vi "HSSS encode.vi"(10 "Crew Status":bool[](array[boolean]), 11 "Array":dbl[](array[numeric])=[111.12345886230469, 111.12345886230469, 111.12345886230469, 9199.099609375, 9299.2001953125, 9399.5, 9499.599609375, 9599.7001953125, 9699.7998046875, 9799.900390625] format="%#.8g") -> (3 "Power string":string)   [LabVIEW 2021]
panel:
  out "length 3":i32
  out "length 2":i32
  out "length":i32
  in  "Array 2":dbl[](array[numeric])=[0.0, 0.0, 0.0, 0.0, 0.0, 0.0, 0.0, 0.0, 0.0, 0.0]
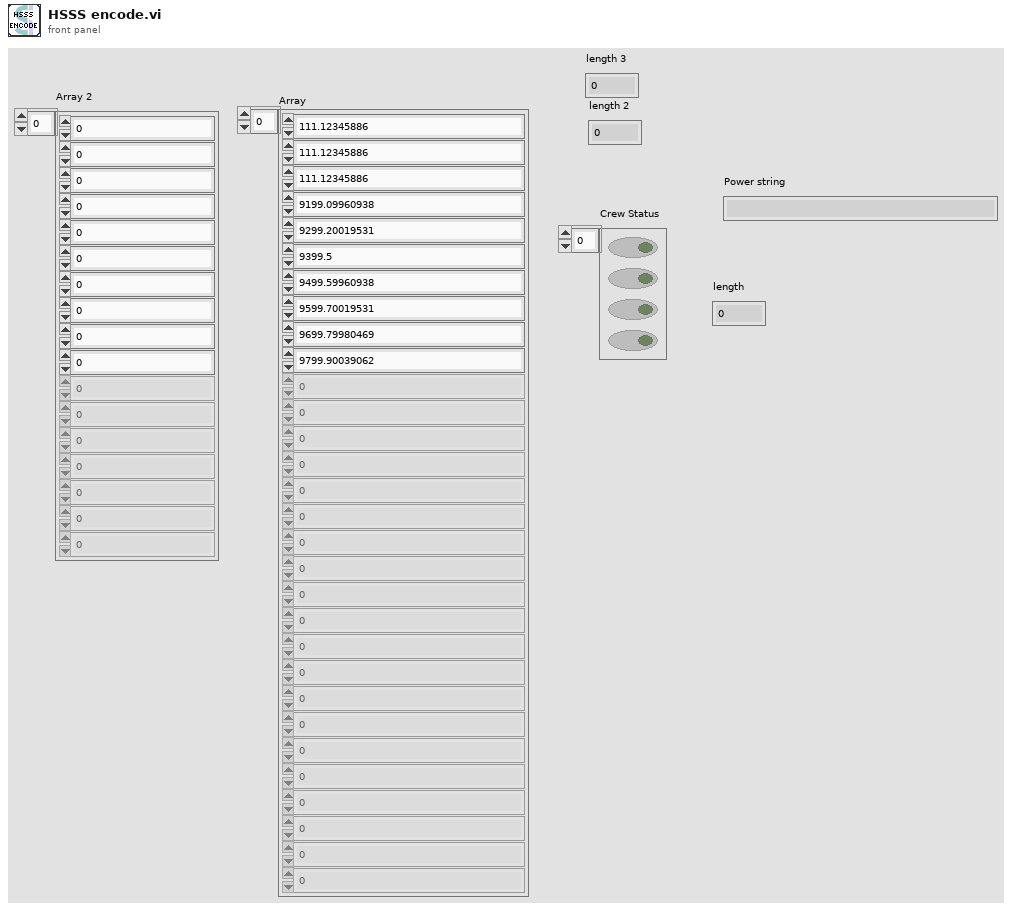
[diagram p1: front panel]
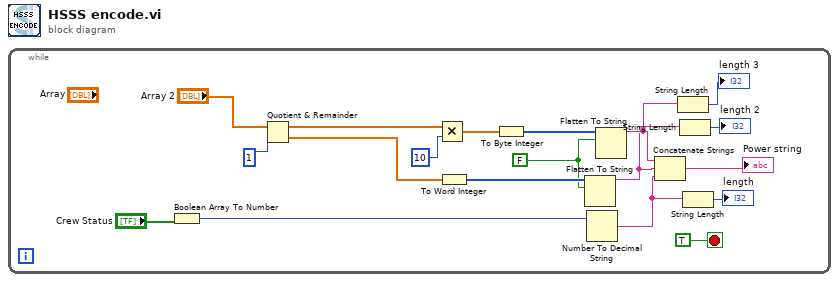
[diagram p0: block diagram]
diagram:
  n1 = while {
    stop <- TRUE stop-if-true
    w11 = FALSE ("prepend array or string size? (T)")
    n2 = Boolean Array To Number(Boolean array="Crew Status") -> (number=w8:u32)
    n3 = Quotient & Remainder(x="Array 2", y=1) -> (x-y*floor(x/y)=w18:dbl[], floor(x/y)=w15:dbl[])
    n4 = Multiply(x=w18, y=10) -> (x*y=w16:dbl[])
    n5 = To Word Integer(number=w15) -> (16bit integer=w14:i16[])
    n6 = To Byte Integer(number=w16) -> (8bit integer=w13:i8[])
    n7 = Flatten To String(anything=w14, prepend array or string size? (T)=w11) -> (data string=w6:string)  [unwired: 2 in, 2 out]
    n8 = Number To Decimal String(number=w8) -> (decimal integer string=w5:string)  [unwired: 1 in]
    n9 = Flatten To String(anything=w13, prepend array or string size? (T)=w11) -> (data string=w7:string)  [unwired: 2 in, 2 out]
    n10 = Concatenate Strings(w7, w6, w5) -> (→"Power string":string)
    n11 = String Length(string=w7) -> (length=→"length 3":i32)
    n12 = String Length(string=w6) -> (length=→"length 2":i32)
    n13 = String Length(string=w5) -> (length=→"length":i32)
  }
